vi "TAT_Manual.vi"(8 "error In":errorcluster) -> (0 "error out":errorcluster)   [LabVIEW 2017]
uses:
  <vilib>/addons/database/Connection.llb/Conn ObjectReference.ctl
  Controls/Ass. Loop Control.ctl
  <vilib>/Utility/error.llb/DialogType.ctl
  <vilib>/Instr/_visa.llb/VISA Configure Serial Port (Instr).vi
  <vilib>/addons/database/NI_Database_API.lvlib
  <vilib>/Utility/config.llb/NI_LVConfig.lvlib
  <vilib>/addons/database/Connection.llb/DB Tools Open Connec (Path).vi
panel:
  out "PREVIOUS BARCODE\nserial no":string[](array[string])
  in  "temp":refnum<visa-resource-name>
  out "array":string[](array[string])
  out "BARCODE STATION 3":string caption="BARCODE:-"
  out "LEAK UNIT RESULT 2":bool caption="LEAK RESULT:-"
  out "LEAK ACTUAL VALUE 2":string
  out "LEAK MAX 2":string
  out "LEAK MIN 2":string
  out "LEAK UNIT RESULT":bool caption="LEAK RESULT:-"
  out "LEAK ACTUAL VALUE":string
  out "LEAK MAX":string
  out "LEAK MIN":string
  out "PREVIOUS BARCODE":string[](array[string])
  out "scanned":string
  out "Scanned Qyt":string
  out "PROJECT :-":string
  out "PACKAGE Qty":string
  out "TORISHI CODE:-":string
  out "PART No.:-":string
  in  "Stop":bool
  out "BARCODE STATION 2":string caption="BARCODE:-"
  out "RESULT STATION 1":bool caption="FINAL RESULT:-"
  out "USER:-":string
  out "PART NAME :-":string
  in  "ASS-Alarms":bool
  out "CYCLE STATUS STATION 1":string caption="CYCLE STATUS:-"
  out "DATE/TIME":string
  # "KAPSE SONS ROBOTICS\n& AUTOMATION"
  # "MANUAL CYCLE"
  # "PACKAGING SLIP"
  # "SCANNED QUANTITY"
  # "PACKAGE QUANTITY"
  # "PREVIOUS BARCODE"
  # "Nm"
  # "POKA-YOKE STATUS"
  # "LEAK TESTING PARAMETER"
  # "MIN"
  # "MAX"
  # "ACTUAL VALUE"
  # "RESULT"
  # "LEAK UNIT"
  # "LEAK PRESSURE"
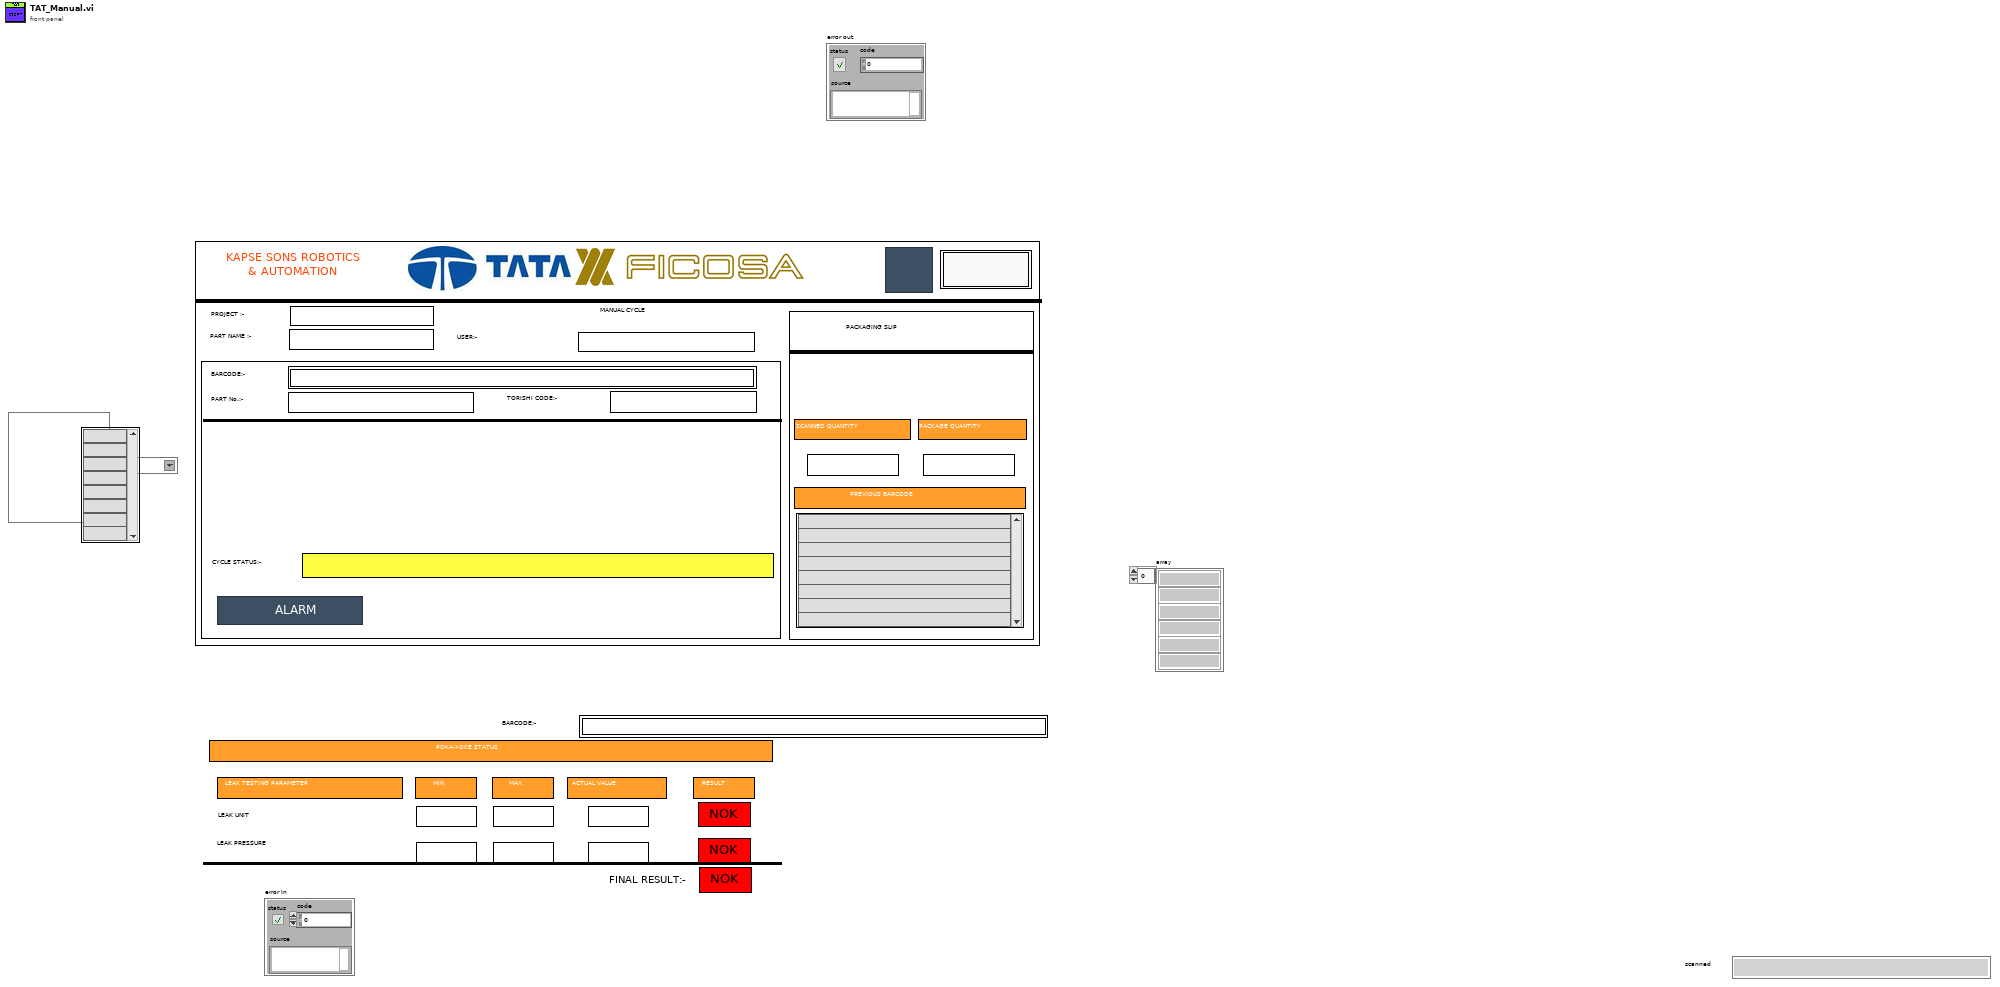
[diagram p1: front panel]
types:
  T1 = typedef "Ass. Loop Control.ctl" = enum16{"Package_Qty_Count", "GENERATE_QR_PRNT", "Cluster_update", "Waiting_for_scan", "barcode CHECK", "Int", "SaveReport ", "Barcode Print", "Start Cycle", "Wait", "Cycle End", "Stop"}
  T2 = typedef "DialogType.ctl" = u16
  T3 = typedef "NI_Database_API.lvlib/Conn ObjectReference.ctl" = refnum<k1>
  T4 = cluster{"Varient number":u16, "Part name":string, "Barcode":string, "connection reference":T3, "Batch_Size":u16, "PART_NO":string, "TORISHI_CODE":string, "scanner com":refnum<visa-resource-name>, "Part Name List":string[], "Varient path":path, "Current Varient path":path, "Communication path":path, "PRN path":path, "printer":refnum<k5>}
  T5 = enum32{"invalid app kind", "Development System", "Run Time System", "Student Edition", "Embedded LabVIEW", "Evaluation", "Custom"}
  T6 = typedef "NI_LVConfig.lvlib/Config Data RefNum.ctl" = refnum<k1>
  T7 = cluster{"seconds since 1Jan1904":timestamp, "Part name":string, "BARCODE STATION 2":string, "table":string, "table":string}
  T8 = cluster{"date string":string, "time string":string, "Part name":string, "PART_NO":string, "TORISHI_CODE":string, "table":string, "table":string, string}
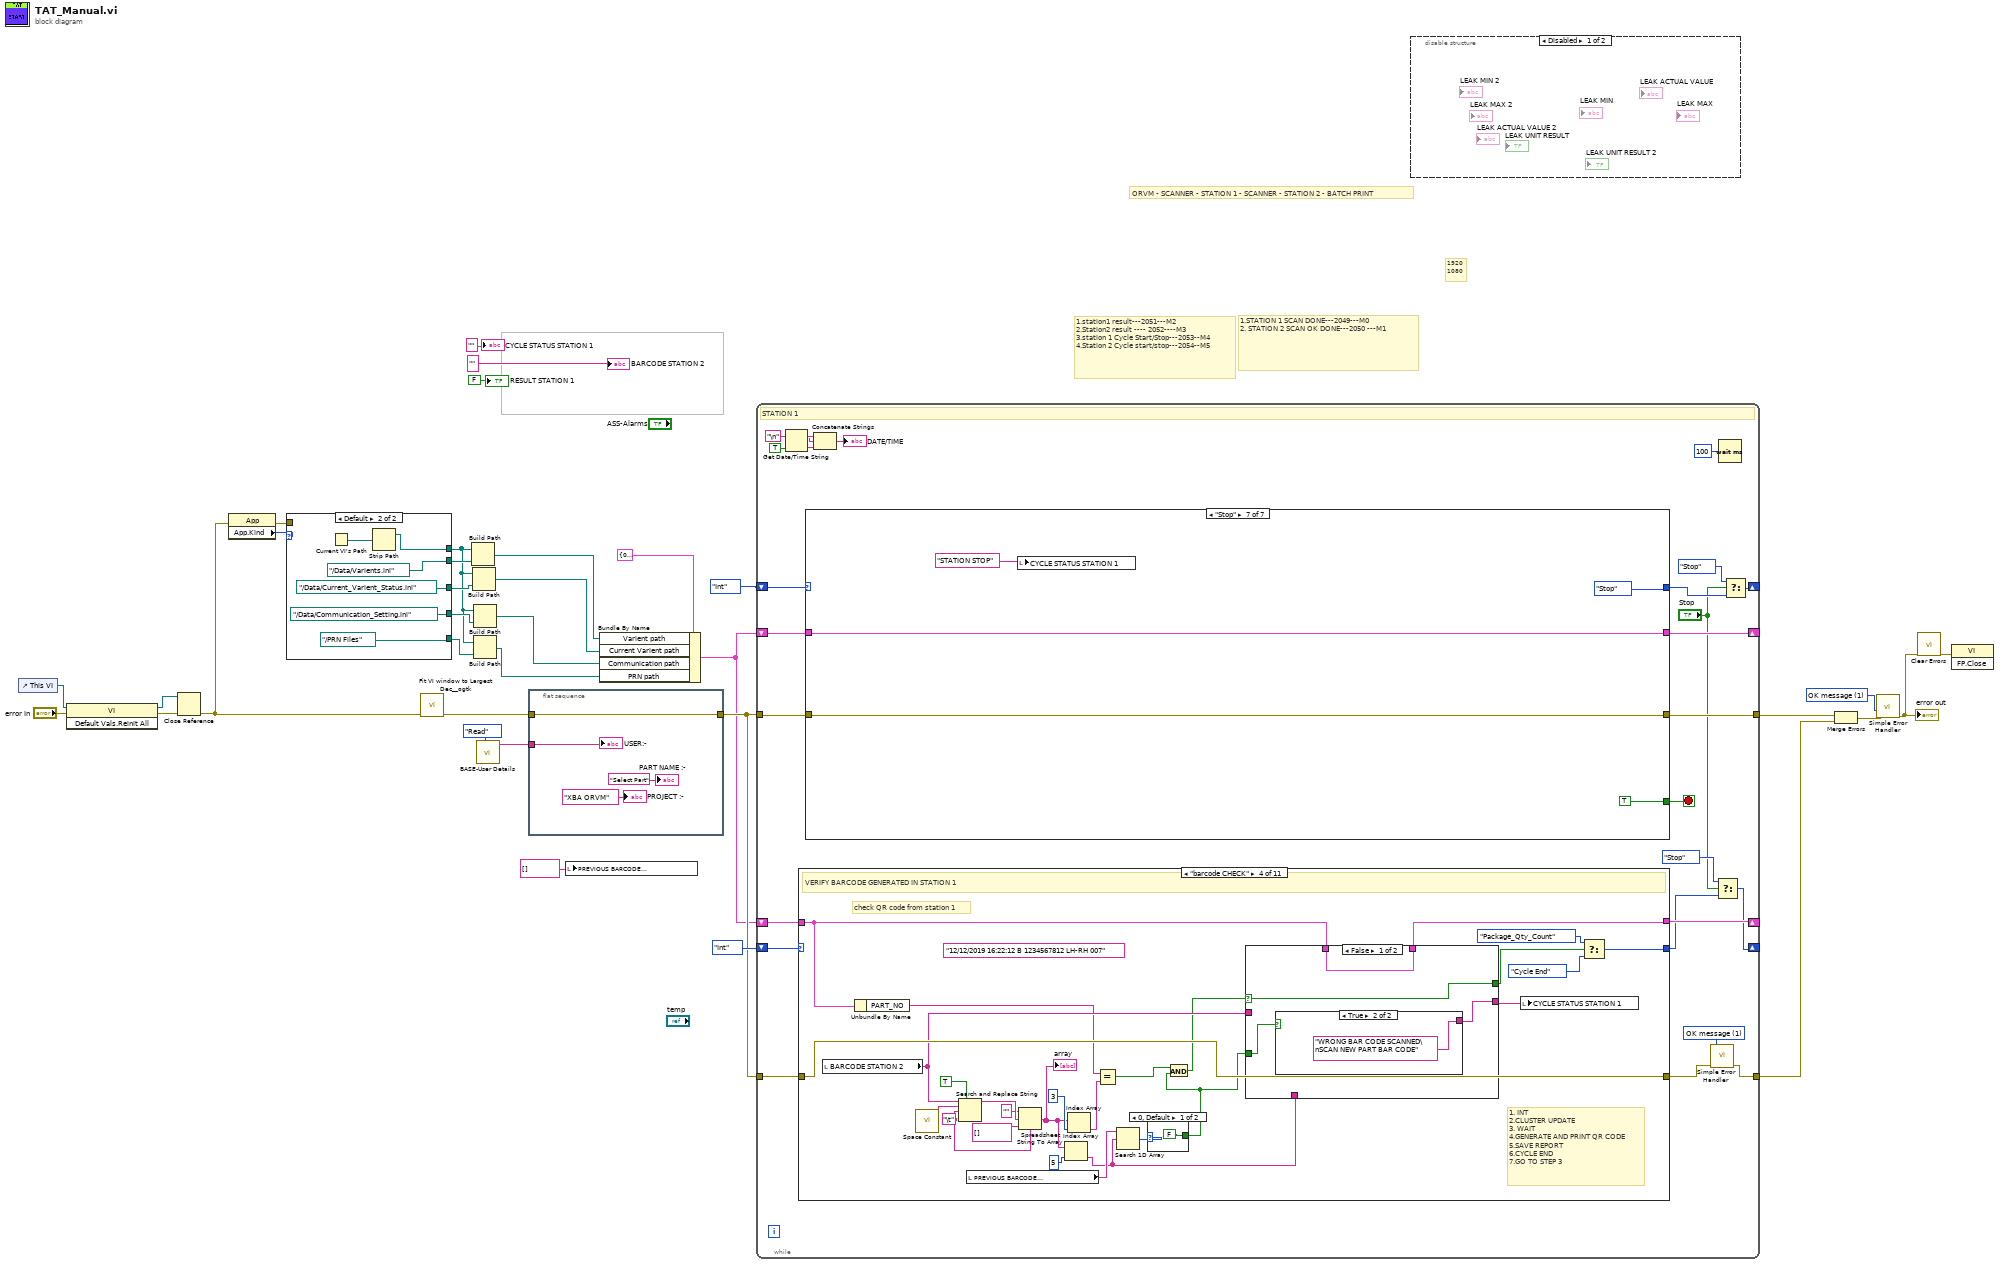
[diagram p0: block diagram]
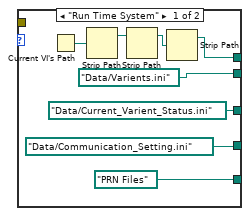
[diagram p2: hidden frame]
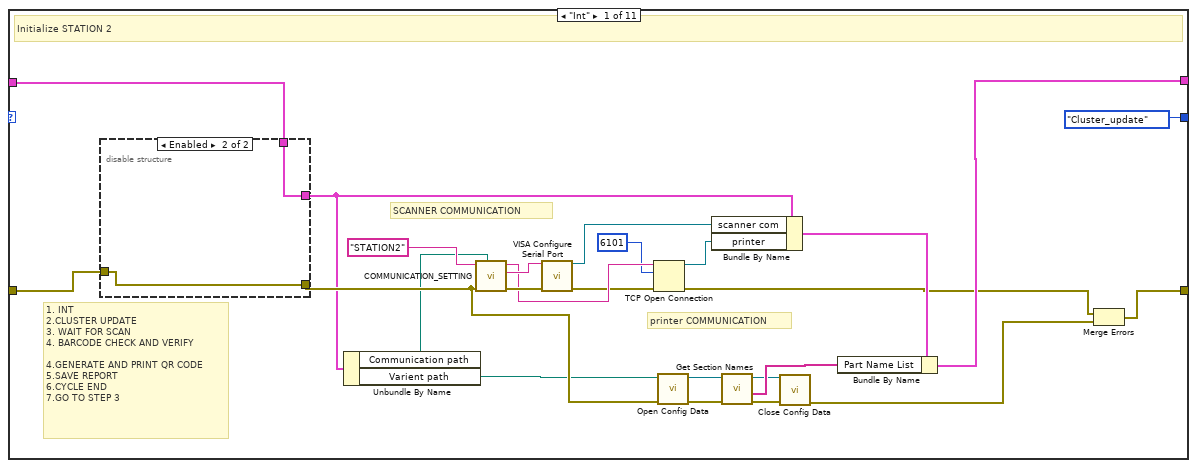
[diagram p4: hidden frame]
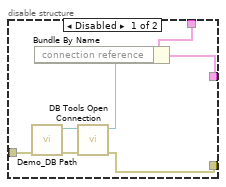
[diagram p5: hidden frame]
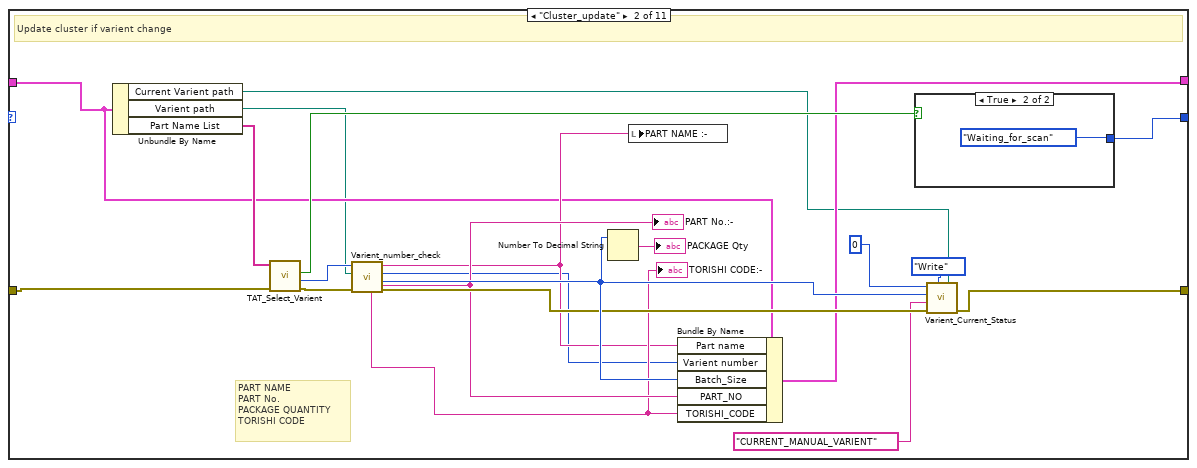
[diagram p6: hidden frame]
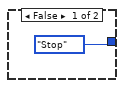
[diagram p7: hidden frame]
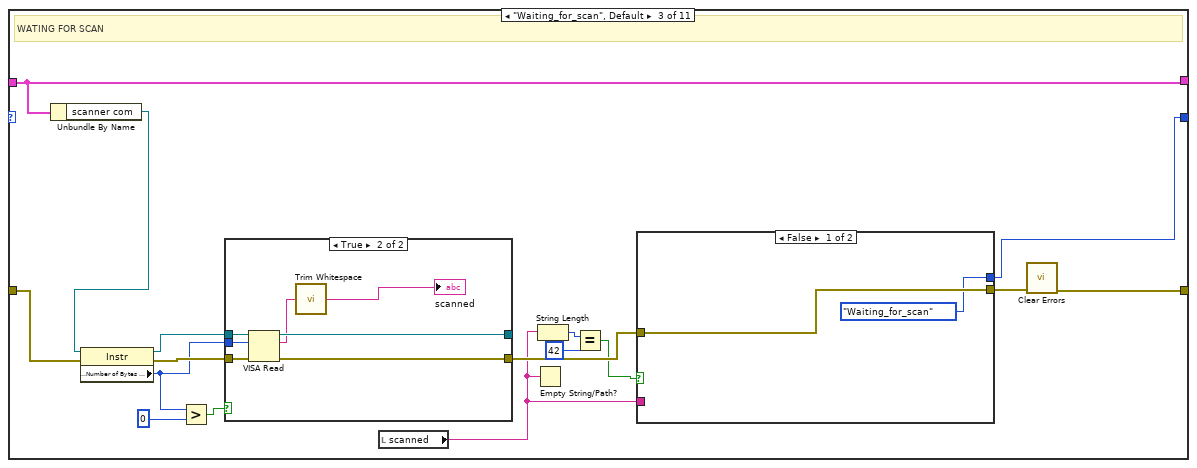
[diagram p8: hidden frame]
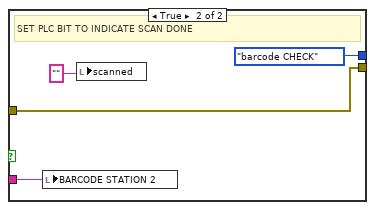
[diagram p10: hidden frame]
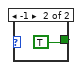
[diagram p11: hidden frame]
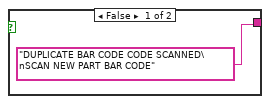
[diagram p12: hidden frame]
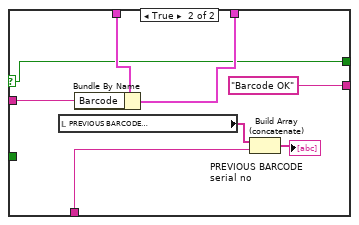
[diagram p13: hidden frame]
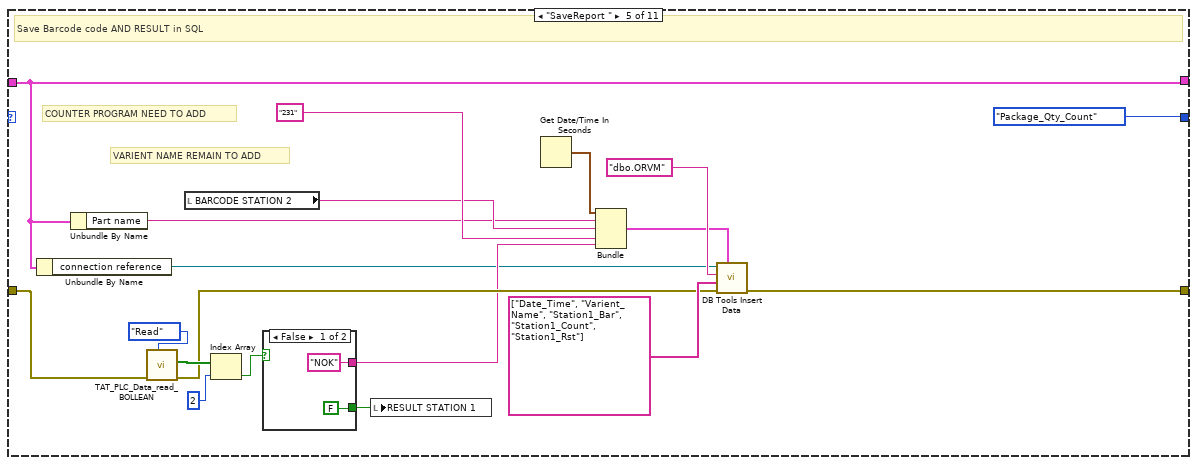
[diagram p14: hidden frame]
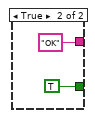
[diagram p15: hidden frame]
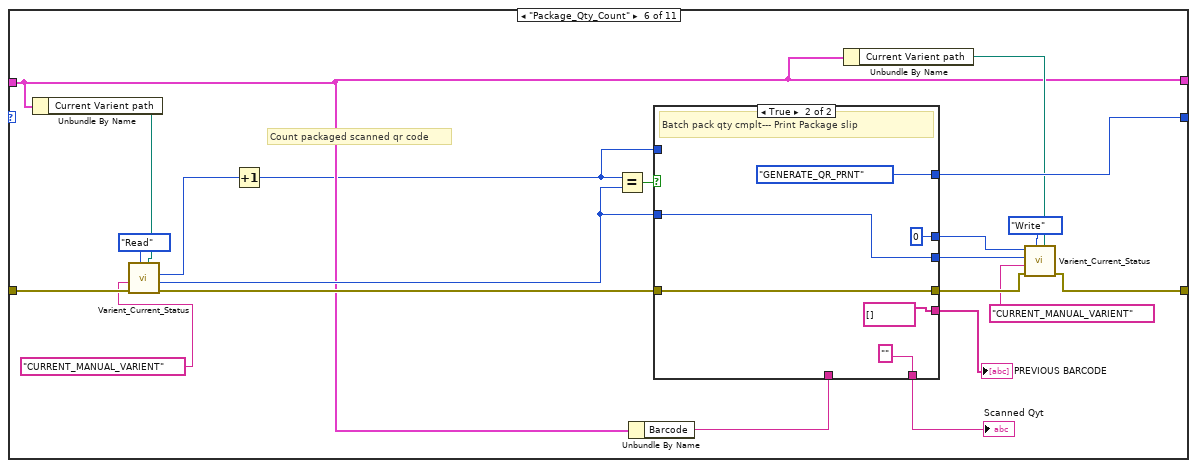
[diagram p16: hidden frame]
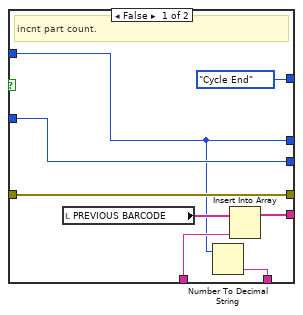
[diagram p17: hidden frame]
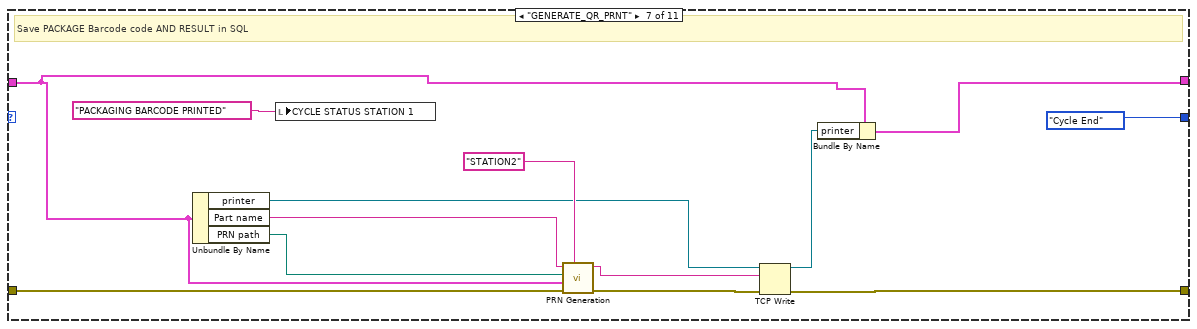
[diagram p18: hidden frame]
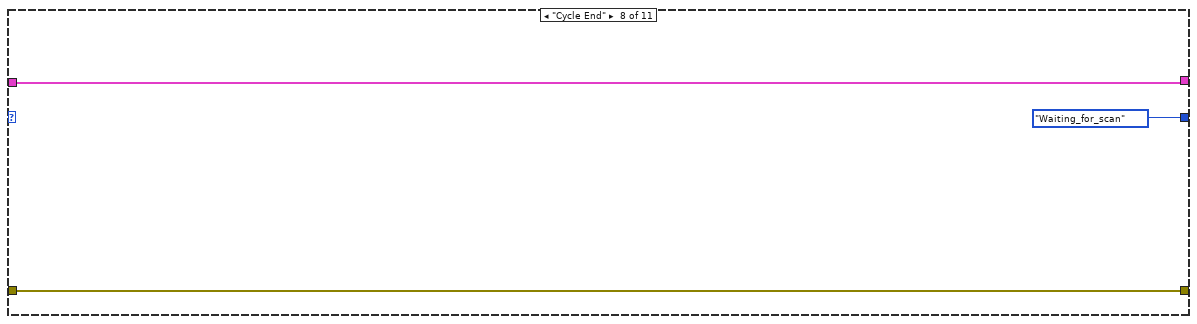
[diagram p19: hidden frame]
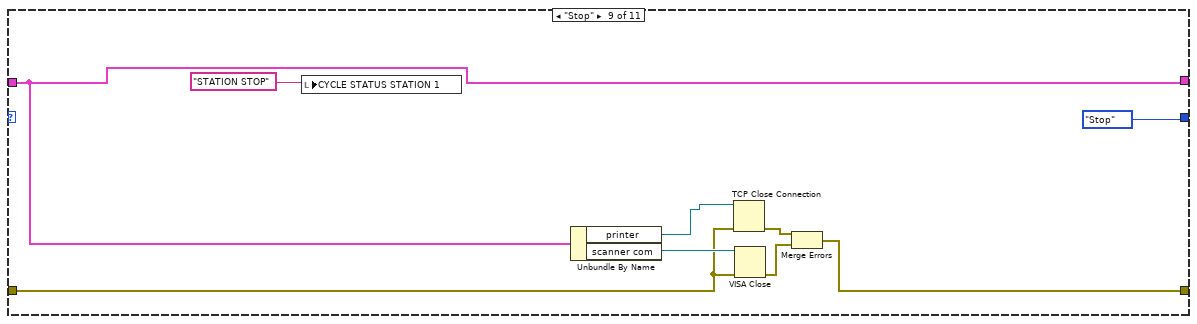
[diagram p20: hidden frame]
diagram:
  w19 = T2 1 items=["no dialog", "OK message", "continue or stop message", "OK message + warnings", "continue/stop + warnings"] ("type of dialog (OK msg:1)")
  # "1920\n1080"
  # "1.STATION 1 SCAN DONE---2049---M0\n2. STATION 2 SCAN OK DONE---2050 ---M1"
  # "1.station1 result---2051---M2\n2.Station2 result ---- 2052----M3\n3.station 1 Cycle Start/Stop---2053--M4\n4.Station 2 Cycle start/stop---2054--M5"
  # "ORVM - SCANNER - STATION 1 - SCANNER - STATION 2 - BATCH PRINT"
  n1 = control-ref of="This VI"() -> (w34:refnum<vi>)
  n2 = invoke class="VI" method="Default Vals.Reinit All"(reference=w34, error in="error In") -> (reference out=w31:refnum<vi>, error out=w32:errorcluster)  [unwired: 1 in, 1 out]
  n3 = Close Reference(reference=w31, error in (no error)=w32) -> (error out=w13:errorcluster)
  n4 = property class="App"(error in=w13) -> (error out=w2:errorcluster, "App.Kind"=w15:T5)  [unwired: 1 in, 1 out]
  n5 = case shown="Default" w15 {
    tunnel: [path "Data/Varients.ini" ("path") path "../Data/Varients.ini" ("path")] -> w14
    tunnel: [w38 w46] -> w4
    tunnel: [path "Data/Current_Varient_Status.ini" ("path") path "../Data/Current_Varient_Status.ini" ("path")] -> w8
    tunnel: [path "Data/Communication_Setting.ini" ("path") path "../Data/Communication_Setting.ini" ("path")] -> w7
    tunnel: [path "PRN Files" ("path") path "../PRN Files" ("path")] -> w5
    tunnel: w2 -> [_ _]
    frame "Run Time System" {
      n6 = Current VI's Path() -> (path=w41:path)
      n7 = Strip Path(path=w41) -> (stripped path=w40:path)  [unwired: 1 out]
      n8 = Strip Path(path=w40) -> (stripped path=w39:path)  [unwired: 1 out]
      n9 = Strip Path(path=w39) -> (stripped path=w38:path)  [unwired: 1 out]
    }
    frame Default {
      n10 = Current VI's Path() -> (path=w47:path)
      n11 = Strip Path(path=w47) -> (stripped path=w46:path)  [unwired: 1 out]
    }
  }
  n12 = call <userlib>:"Fit VI window to Largest Dec__ogtk.vi"("error in (no error)"=w13) -> ("error out"=w30:errorcluster)  [unwired: 5 in, 1 out]
  n13 = Build Path(base path=w4, name or relative path=w14) -> (appended path=w10:path)
  n14 = Build Path(base path=w4, name or relative path=w8) -> (appended path=w9:path)
  n15 = Build Path(base path=w4, name or relative path=w7) -> (appended path=w6:path)
  n16 = Build Path(base path=w4, name or relative path=w5) -> (appended path=w3:path)
  n17 = call "BASE-User Details.vi"("Enum"=enum16{"Read", "Write"}."Read") -> ("User Name Out"=w20:string)  [unwired: 9 in, 1 out]
  n18 = flat-sequence {
    tunnel: [w52] -> w17
    tunnel: w30 -> [w52]
    tunnel: w20 -> [w51]
    frame #0 {
      "USER:-" <- w51
      "PART NAME :-" <- "Select Part"
      "PROJECT :-" <- "XBA ORVM" ("PROJECT")
    }
  }
  n19 = local write "PREVIOUS BARCODE\nserial no"(string[] [] ("PREVIOUS BARCODE\nserial no")) -> ()
  n20 = Bundle By Name(cluster=T4 {"Varient number"=0, "Part name"="", "Barcode"="", "connection reference"=refnum, "Batch_Size"=0, "PART_NO"="", "TORISHI_CODE"="", "scanner com"="", "Part Name List"=[], "Varient path"=path "", "Current Varient path"=path "", "Communication path"=path "", "PRN path"=path "", "printer"=refnum}, "Varient path"=w10, "Current Varient path"=w9, "Communication path"=w6, "PRN path"=w3) -> (w11:T4)
  n21 = while {
    tunnel: w17 -> [w73]
    shift-right: [w72] -> _
    shift-left: Ass._Loop_Control."Int" ("Enum") -> [w78]
    shift-right: [w76] -> _
    shift-left: w11 -> [w75]
    tunnel: [w74] -> w26
    shift-right: [w58] -> _
    shift-left: Ass._Loop_Control."Int" ("Enum") -> [w63]
    tunnel: w17 -> [w62]
    shift-right: [w60] -> _
    shift-left: w11 -> [w61]
    tunnel: [w53] -> w16
    stop <- w64 stop-if-true
    w55 = T2 1 items=["no dialog", "OK message", "continue or stop message", "OK message + warnings", "continue/stop + warnings"] ("type of dialog (OK msg:1)")
    # "STATION 1"
    n22 = Get Date/Time String(want seconds? (F)=TRUE) -> (date string=w68:string, time string=w67:string)  [unwired: 2 in]
    n23 = case shown="\"barcode CHECK\"" w63 {
      tunnel: [Ass._Loop_Control."Cluster_update" ("Enum") w115 w145 w192 Ass._Loop_Control."Package_Qty_Count" ("Enum") w241 Ass._Loop_Control."Cycle End" ("Enum") Ass._Loop_Control."Waiting_for_scan" ("Enum") Ass._Loop_Control."Stop" ("Enum") Ass._Loop_Control."Wait" ("Enum") Ass._Loop_Control."Wait" ("Enum")] -> w57
      tunnel: [w89 w117 w144 w189 w211 w237 w269 w280 w287 w294 w295] -> w60
      tunnel: [w88 w120 w151 w188 w210 w246 w272 w281 w288 w292 w296] -> w54
      tunnel: w62 -> [w98 w119 w146 w188 w209 w252 w275 w281 w285 w292 w296]
      tunnel: w61 -> [w97 w118 w144 w190 w211 w237 w267 w280 w287 w294 w295]
      frame "Int" {
        # "1. INT\n2.CLUSTER UPDATE\n3. WAIT FOR SCAN\n4. BARCODE CHECK AND VERIFY\n\n4.GENERATE AND PRINT QR CODE\n5.SAVE REPORT\n6.CYCLE END\n7.GO TO STEP 3"
        # "printer COMMUNICATION"
        # "SCANNER COMMUNICATION"
        # "Initialize STATION 2"
        n24 = disable-structure shown="Enabled" {
          disable-tunnel: [w109 w112] -> w86
          disable-tunnel: [w107 w111] -> w87
          disable-tunnel: w98 -> [w105 w111]
          disable-tunnel: w97 -> [w104 w112]
          frame Disabled {
            n25 = call "Demo_DB Path.vi"("error in"=w105) -> ("error out"=w108:errorcluster, "DB Path"=w110:path)  [unwired: 9 in]
            n26 = call-poly <vilib>:"DB Tools Open Connection.vi"("error in (no error)"=w108, "connection information"=w110) -> ("error out"=w107:errorcluster, "connection reference"=w106:T3)  [unwired: 6 in]
            n27 = Bundle By Name(cluster=w104, "connection reference"=w106) -> (w109:T4)
          }
          frame Enabled {
          }
        }
        n28 = Unbundle By Name(w86) -> ("Communication path"=w84:path, "Varient path"=w85:path)
        n29 = call "COMMUNICATION_SETTING.vi"("communication path"=w84, "error in"=w87, "STATION"="STATION2") -> ("error out"=w102:errorcluster, "SCAN_COM"=w99:string, "PRINT_COM"=w83:string)  [unwired: 6 in]
        n30 = call-poly "VISA Configure Serial Port"("VISA resource name"=w99, "error in (no error)"=w102) -> ("VISA resource name out"=w100:refnum<visa-resource-name>, "error out"=w82:errorcluster)  [unwired: 12 in]
        n31 = TCP Open Connection(address=w83, remote port or service name=u16 6101, error in (no error)=w82) -> (connection ID=w80:refnum<k5>, error out=w81:errorcluster)  [unwired: 2 in]
        n32 = call <vilib>:"Open Config Data.vi"("error in (no error)"=w87, "configuration file path"=w85) -> ("error out"=w94:errorcluster, "refnum"=w95:T6)  [unwired: 7 in, 1 out]
        n33 = Bundle By Name(cluster=w86, "scanner com"=w100, "printer"=w80) -> (w90:T4)
        n34 = call <vilib>:"Get Section Names.vi"("error in (no error)"=w94, "refnum"=w95) -> ("error out"=w93:errorcluster, "section names"=w96:string[], "refnum out"=w92:T6)  [unwired: 7 in]
        n35 = call <vilib>:"Close Config Data.vi"("error in (no error)"=w93, "refnum"=w92) -> ("error out"=w91:errorcluster)  [unwired: 8 in, 1 out]
        n36 = Bundle By Name(cluster=w90, "Part Name List"=w96) -> (w89:T4)
        n37 = Merge Errors(w81, w91) -> (w88:errorcluster)
      }
      frame "Cluster_update" {
        # "PART NAME\nPART No.\nPACKAGE QUANTITY\nTORISHI CODE"
        # "Update cluster if varient change"
        n38 = Unbundle By Name(w118) -> ("Current Varient path"=w113:path, "Varient path"=w114:path, "Part Name List"=w130:string[])
        n39 = call "TAT_Select_Varient.vi"("Part List"=w130, "Error In"=w119) -> ("Cancle"=w133:bool, "Varient no"=w131:i32, "error out"=w132:errorcluster)  [unwired: 5 in, 1 out]
        n40 = call "Varient_number_check.vi"("error in"=w132, "Varient path"=w114, "Varient No."=w131) -> ("error out"=w128:errorcluster, "Batch Size"=w129:i32, "Varient Number"=w123:i32, "Part Name"=w124:string, "PART_NO"=w127:string, "TORISHI_CODE"=w126:string)  [unwired: 3 in]
        "PART No.:-" <- w127
        "TORISHI CODE:-" <- w126
        n41 = Number To Decimal String(number=w129) -> (decimal integer string=→"PACKAGE Qty":string)  [unwired: 1 in]
        n42 = local write "PART NAME :-"(w124) -> ()
        n43 = Bundle By Name(cluster=w118, "Part name"=w124, "Varient number"=w123, "Batch_Size"=w129, "PART_NO"=w127, "TORISHI_CODE"=w126) -> (w117:T4)
        n44 = case shown="True" w133 {
          tunnel: [Ass._Loop_Control."Stop" ("Enum") Ass._Loop_Control."Waiting_for_scan" ("Enum")] -> w115
          frame False {
          }
          frame True {
          }
        }
        n45 = call "Varient_Current_Status.vi"("Currenrt Varient path"=w113, "Enum"=enum16{"Write", "Read"}."Write", "error in"=w128, "AUTO/MANUAL"="CURRENT_MANUAL_VARIENT", "Batch Size"=w129, "Varient count"=0) -> ("error out"=w120:errorcluster)  [unwired: 3 in, 2 out]
      }
      frame "Waiting_for_scan", Default {
        # "WATING FOR SCAN"
        n46 = Unbundle By Name(w144) -> ("scanner com"=w143:refnum<visa-resource-name>)
        n47 = property class="Instr"(reference=w143, error in=w146) -> (reference out=w150:refnum<visa-resource-name>, error out=w149:errorcluster, "Serial Settings:Number of Bytes at Serial Port"=w142:u32)
        n48 = Greater?(x=w142, y=u32 0) -> (0:w141:bool)
        n49 = case shown="True" w141 {
          tunnel: w150 -> [w153 w160]
          tunnel: w149 -> [w152 w159]
          tunnel: w142 -> [_ w158]
          tunnel: [w153 w157] -> _
          tunnel: [w152 w154] -> w148
          frame False {
          }
          frame True {
            n50 = VISA Read(VISA resource name=w160, byte count=w158, error in (no error)=w159) -> (VISA resource name out=w157:refnum<visa-resource-name>, read buffer=w155:string, error out=w154:errorcluster)  [unwired: 1 out]
            n51 = call <vilib>:"Trim Whitespace.vi"("string"=w155) -> ("trimmed string"=→"scanned":string)  [unwired: 1 in]
          }
        }
        n52 = local read "scanned"() -> (w139:string)
        n53 = Empty String/Path?(string/path=w139) -> ()  [unwired: 1 out]
        n54 = String Length(string=w139) -> (length=w138:i32)
        n55 = Equal?(x=w138, y=42) -> (x = y?=w136:bool)
        n56 = case shown="False" w136 {
          tunnel: w148 -> [w162 w166]
          tunnel: [w162 w166] -> w147
          tunnel: w139 -> [_ w165]
          tunnel: [Ass._Loop_Control."Waiting_for_scan" ("Enum") Ass._Loop_Control."barcode CHECK" ("Enum")] -> w145
          frame False {
          }
          frame True {
            # "SET PLC BIT TO INDICATE SCAN DONE"
            n57 = local write "BARCODE STATION 2"(w165) -> ()
            n58 = local write "scanned"("") -> ()
          }
        }
        n59 = call <vilib>:"Clear Errors.vi"("error in (no error)"=w147) -> ("error out"=w151:errorcluster)  [unwired: 5 in, 1 out]
      }
      frame "barcode CHECK" {
        w181 = "\t"
        (unwired) "12/12/2019 16:22:12 B 1234567812 LH-RH 007" ("string")
        # "check QR code from station 1"
        # "1. INT\n2.CLUSTER UPDATE\n3. WAIT\n4.GENERATE AND PRINT QR CODE\n5.SAVE REPORT\n6.CYCLE END\n7.GO TO STEP 3"
        # "VERIFY BARCODE GENERATED IN STATION 1"
        n60 = local read "BARCODE STATION 2"() -> (w178:string)
        n61 = Unbundle By Name(w190) -> ("PART_NO"=w176:string)
        n62 = call <vilib>:"Space Constant.vi"() -> ("String"=w184:string)
        n63 = Search and Replace String(replace all?=TRUE ("replace all? (F)"), input string=w178, search string=w184, replace string=w181) -> (result string=w182:string)  [unwired: 4 in, 3 out]
        n64 = local read "PREVIOUS BARCODE\nserial no"() -> (w168:string[])
        n65 = Spreadsheet String To Array(delimiter (Tab)=w181, format string="", spreadsheet string=w182, array type (2D Dbl)=string[] []) -> (array=w169:string[])
        "array" <- w169
        n66 = Index Array(array=w169, index=5) -> (element=w167:string)
        n67 = Index Array(array=w169, index=3) -> (element=w175:string)
        n68 = Equal?(x=w176, y=w175) -> (x = y?=w173:bool)
        n69 = Search 1D Array(1D array=w168, element=w167) -> (index of element=w174:i32)  [unwired: 1 in]
        n70 = case shown="0, Default" w174 {
          tunnel: [FALSE TRUE] -> w171
          frame 0, Default {
          }
          frame -1 {
          }
        }
        n71 = And(x=w173, y=w171) -> (x .and. y?=w172:bool)
        n72 = case shown="False" w172 {
          selector: w172 -> [w196 w204]
          tunnel: [w198 "Barcode OK" ("Cycle Status")] -> w191
          tunnel: w190 -> [w197 w207]
          tunnel: [w197 w206] -> w189
          tunnel: w178 -> [_ w205]
          tunnel: [w196 w204] -> w185
          tunnel: w171 -> [w195 _]
          tunnel: w167 -> [_ w202]
          frame False {
            n73 = case shown="True" w195 {
              tunnel: ["DUPLICATE BAR CODE CODE SCANNED\nSCAN NEW PART BAR CODE" ("Cycle Status") "WRONG BAR CODE SCANNED\nSCAN NEW PART BAR CODE" ("Cycle Status")] -> w198
              frame False {
              }
              frame True {
              }
            }
          }
          frame True {
            n74 = local read "PREVIOUS BARCODE\nserial no"() -> (w201:string[])
            n75 = Bundle By Name(cluster=w207, "Barcode"=w205) -> (w206:T4)
            n76 = Build Array (concatenate)(w201, w202) -> (→"PREVIOUS BARCODE\nserial no":string[])
          }
        }
        n77 = local write "CYCLE STATUS STATION 1"(w191) -> ()
        n78 = Select(t=Ass._Loop_Control."Package_Qty_Count" ("Enum"), s=w185, f=Ass._Loop_Control."Cycle End" ("Enum")) -> (s? t:f=w192:T1)
      }
      frame "SaveReport " {
        # "COUNTER PROGRAM NEED TO ADD"
        # "VARIENT NAME REMAIN TO ADD"
        # "Save Barcode code AND RESULT in SQL"
        n79 = Unbundle By Name(w211) -> ("connection reference"=w212:T3)
        n80 = Unbundle By Name(w211) -> ("Part name"=w220:string)
        n81 = call "TAT_PLC_Data_read_BOLLEAN.vi"("Enum"=enum16{"Read", "Write"}."Read", "error in (no error)"=w209) -> ("error out"=w217:errorcluster, "Array 2"=w218:bool[])  [unwired: 8 in]
        n82 = local read "BARCODE STATION 2"() -> (w221:string)
        n83 = Index Array(array=w218, index=2) -> (element=w214:bool)
        n84 = case shown="False" w214 {
          tunnel: ["NOK" ("table") "OK" ("table")] -> w215
          tunnel: [FALSE TRUE] -> w213
          frame False {
          }
          frame True {
          }
        }
        n85 = local write "RESULT STATION 1"(w213) -> ()
        n86 = Get Date/Time In Seconds() -> (seconds since 1Jan1904=w222:timestamp)
        n87 = Bundle("seconds since 1Jan1904"=w222, "Part name"=w220, "BARCODE STATION 2"=w221, "table"="231", "table"=w215) -> (w225:T7)  [unwired: 1 in]
        n88 = call <vilib>:"DB Tools Insert Data.vi"("data"=w225, "error in (no error)"=w217, "columns"=string[] ["Date_Time", "Varient_Name", "Station1_Bar", "Station1_Count", "Station1_Rst"] ("columns 2"), "table"="dbo.ORVM", "connection reference"=w212) -> ("error out"=w210:errorcluster)  [unwired: 5 in, 1 out]
      }
      frame "Package_Qty_Count" {
        # "Count packaged scanned qr code"
        n89 = Unbundle By Name(w237) -> ("Current Varient path"=w236:path)
        n90 = call "Varient_Current_Status.vi"("Currenrt Varient path"=w236, "Enum"=enum16{"Write", "Read"}."Read", "error in"=w252, "AUTO/MANUAL"="CURRENT_MANUAL_VARIENT") -> ("error out"=w250:errorcluster, "Batch Size"=w244:i32, "Varient Count"=w249:i32)  [unwired: 5 in]
        n91 = Increment(x=w249) -> (x+1=w235:i32)
        n92 = Equal?(x=w235, y=w244) -> (x = y?=w248:bool)
        n93 = Unbundle By Name(w237) -> ("Barcode"=w234:string)
        n94 = case shown="True" w248 {
          tunnel: [w260 w266] -> w245
          tunnel: w250 -> [w260 w266]
          tunnel: w235 -> [w253 _]
          tunnel: w244 -> [w259 w265]
          tunnel: [w259 w265] -> w243
          tunnel: [w253 0] -> w242
          tunnel: [Ass._Loop_Control."Cycle End" ("Enum") Ass._Loop_Control."GENERATE_QR_PRNT" ("Enum")] -> w241
          tunnel: w234 -> [w256 _]
          tunnel: [w255 string[] [] ("PREVIOUS BARCODE")] -> w233
          tunnel: [w254 ""] -> w232
          frame False {
            # "incnt part count."
            n95 = local read "PREVIOUS BARCODE"() -> (w257:string[])
            n96 = Number To Decimal String(number=w253) -> (decimal integer string=w254:string)  [unwired: 1 in]
            n97 = Insert Into Array(array=w257, new element=w256) -> (w255:string[])  [unwired: 1 in]
          }
          frame True {
            # "Batch pack qty cmplt--- Print Package slip"
          }
        }
        "PREVIOUS BARCODE" <- w233
        "Scanned Qyt" <- w232
        n98 = Unbundle By Name(w237) -> ("Current Varient path"=w238:path)
        n99 = call "Varient_Current_Status.vi"("Currenrt Varient path"=w238, "Enum"=enum16{"Write", "Read"}."Write", "error in"=w245, "AUTO/MANUAL"="CURRENT_MANUAL_VARIENT", "Batch Size"=w243, "Varient count"=w242) -> ("error out"=w246:errorcluster)  [unwired: 3 in, 2 out]
      }
      frame "GENERATE_QR_PRNT" {
        # "Save PACKAGE Barcode code AND RESULT in SQL"
        n100 = Unbundle By Name(w267) -> ("printer"=w271:refnum<k5>, "Part name"=w276:string, "PRN path"=w273:path)
        n101 = local write "CYCLE STATUS STATION 1"("PACKAGING BARCODE PRINTED" ("Cycle Status")) -> ()
        n102 = call "PRN Generation.vi"("FILE NAME"="STATION2", "error in (no error)"=w275, "Cluster"=w267, "PRN path"=w273, "File Folder Name"=w276) -> ("error out"=w277:errorcluster, "PRN to Print"=w270:string)  [unwired: 4 in, 1 out]
        n103 = TCP Write(connection ID=w271, data in=w270, error in (no error)=w277) -> (connection ID out=w268:refnum<k5>, error out=w272:errorcluster)  [unwired: 1 in, 1 out]
        n104 = Bundle By Name(cluster=w267, "printer"=w268) -> (w269:T4)
      }
      frame "Cycle End" {
      }
      frame "Stop" {
        n105 = local write "CYCLE STATUS STATION 1"("STATION STOP" ("Cycle Status")) -> ()
        n106 = Unbundle By Name(w287) -> ("printer"=w284:refnum<k5>, "scanner com"=w286:refnum<visa-resource-name>)
        n107 = TCP Close Connection(connection ID=w284, error in (no error)=w285) -> (error out=w283:errorcluster)  [unwired: 1 in, 1 out]
        n108 = VISA Close(VISA resource name=w286, error in (no error)=w285) -> (error out=w289:errorcluster)
        n109 = Merge Errors(w283, w289) -> (w288:errorcluster)
      }
      frame "Wait" {
        # "Wait-- NOT USED"
      }
      frame "Start Cycle" {
        n110 = local write "CYCLE STATUS STATION 1"("Cycle started" ("Cycle Status")) -> ()
      }
    }
    n111 = case shown="\"Stop\"" w78 {
      tunnel: [Ass._Loop_Control."Cluster_update" ("Enum") Ass._Loop_Control."Wait" ("Enum") Ass._Loop_Control."Wait" ("Enum") Ass._Loop_Control."Wait" ("Enum") Ass._Loop_Control."Cycle End" ("Enum") Ass._Loop_Control."Wait" ("Enum") Ass._Loop_Control."Stop" ("Enum")] -> w71
      tunnel: [w300 w304 w307 w313 w325 w345 w348] -> w76
      tunnel: w75 -> [w300 w304 w307 w313 w325 w345 w348]
      tunnel: [_ _ FALSE _ _ _ TRUE] -> w64
      tunnel: [w299 w305 w308 w310 w335 w344 w346] -> w74
      tunnel: w73 -> [w299 w305 w308 w310 w327 w344 w346]
      frame "Int" {
        # "1. INT\n2.CLUSTER UPDATE\n3. WAIT\n4.\n5.SAVE REPORT\n6.CYCLE END\n7.GO TO STEP 3"
        # "Initialize"
        n112 = local write "CYCLE STATUS STATION 1"("WAIT FOR CYCLE START" ("Cycle Status")) -> ()
      }
      frame "Cluster_update" {
        # "Update cluster if varient change"
      }
      frame "Wait", Default {
        # "WAITING FORM CCYLE TO COMPLE TO PRINT QR"
        # "Wait"
      }
      frame "Start Cycle" {
        n113 = local write "CYCLE STATUS STATION 1"("Cycle started" ("Cycle Status")) -> ()
      }
      frame "SaveReport " {
        (unwired) string[] ["Date", "Time", "Part_Name", "Part_No", "Torishi_Code", "Shift", "Station1_Rst", "Packaging_Qty", "Serial_No", "QR_Code", "Station2_Rst"] ("columns 2")
        # "Save Barcode code AND RESULT in SQL"
        n114 = Unbundle By Name(w325) -> ("connection reference"=w334:T3)
        n115 = Unbundle By Name(w325) -> ("Part name"=w333:string, "PART_NO"=w321:string, "TORISHI_CODE"=w320:string, "Batch_Size"=w317:u16)
        n116 = call "TAT_PLC_Data_read_BOLLEAN.vi"("Enum"=enum16{"Read", "Write"}."Read", "error in (no error)"=w327) -> ("error out"=w330:errorcluster, "Array 2"=w331:bool[])  [unwired: 8 in]
        n117 = Number To Decimal String(number=w317) -> (decimal integer string=w316:string)  [unwired: 1 in]
        n118 = Index Array(array=w331, index=2) -> (element=w328:bool)
        n119 = case shown="False" w328 {
          tunnel: ["NOK" ("table") "OK" ("table")] -> w319
          tunnel: [FALSE TRUE] -> w326
          frame False {
          }
          frame True {
          }
        }
        n120 = local write "RESULT STATION 1"(w326) -> ()
        n121 = Get Date/Time In Seconds() -> (seconds since 1Jan1904=w324:timestamp)
        n122 = Get Date/Time String(seconds (now)=w324) -> (date string=w323:string, time string=w322:string)  [unwired: 2 in]
        n123 = Bundle("date string"=w323, "time string"=w322, "Part name"=w333, "PART_NO"=w321, "TORISHI_CODE"=w320, "table"="SHIFT TO ADD HERE", "table"=w319, w316) -> (w336:T8)  [unwired: 1 in]
        n124 = call <vilib>:"DB Tools Insert Data.vi"("data"=w336, "error in (no error)"=w330, "columns"=string[] ["Date", "Time", "Part_Name", "Part_No", "Torishi_Code", "Shift", "Station1_Rst", "Packaging_Qty"] ("columns 2"), "table"="dbo.XBA_ORVM", "connection reference"=w334) -> ("error out"=w335:errorcluster)  [unwired: 5 in, 1 out]
        n125 = local read "BARCODE STATION 2"() -> (→"BARCODE STATION 3":string)
      }
      frame "Cycle End" {
      }
      frame "Stop" {
        n126 = local write "CYCLE STATUS STATION 1"("STATION STOP" ("Cycle Status")) -> ()
      }
    }
    n127 = Concatenate Strings(w68, "\n", w67) -> (→"DATE/TIME":string)
    n128 = call <vilib>:"Simple Error Handler.vi"("type of dialog (OK msg:1)"=w55, "error in (no error)"=w54) -> ("error out"=w53:errorcluster)  [unwired: 3 in, 4 out]
    n129 = Select(t=Ass._Loop_Control."Stop" ("Enum"), s="Stop", f=w57) -> (s? t:f=w58:T1)
    n130 = Wait (ms)(milliseconds to wait=u32 100) -> ()  [unwired: 1 out]
    n131 = Select(t=Ass._Loop_Control."Stop" ("Enum"), s="Stop", f=w71) -> (s? t:f=w72:T1)
  }
  n132 = disable-structure shown="Disabled" {
    frame Disabled {
    }
    frame Enabled {
    }
  }
  n133 = Merge Errors(w26, w16) -> (w24:errorcluster)
  n134 = call <vilib>:"Simple Error Handler.vi"("type of dialog (OK msg:1)"=w19, "error in (no error)"=w24) -> ("error out"=w23:errorcluster)  [unwired: 3 in, 4 out]
  "error out" <- w23
  n135 = call <vilib>:"Clear Errors.vi"("error in (no error)"=w23) -> ("error out"=w22:errorcluster)  [unwired: 5 in, 1 out]
  n136 = invoke class="VI" method="FP.Close"(error in=w22) -> ()  [unwired: 2 in, 3 out]
  "CYCLE STATUS STATION 1" <- ""
  "BARCODE STATION 2" <- ""
  "RESULT STATION 1" <- FALSE ("want seconds? (F)")
